vi "PPL_DRIVE_Get_Wheel_Speeds.vi"() -> (1 "Right Wheel Speed M/S":dbl format="%17.2f", 3 "Left Wheel Speed M/S":dbl format="%17.2f")   [LabVIEW 2019]
uses:
  PPL_DRIVE_GLOBALS.vi
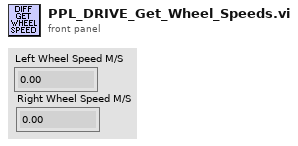
[diagram p1: front panel]
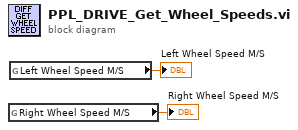
[diagram p0: block diagram]
diagram:
  n1 = global read "PPL_DRIVE_GLOBALS.vi" "Right Wheel Speed M/S"() -> (→"Right Wheel Speed M/S":dbl)
  n2 = global read "PPL_DRIVE_GLOBALS.vi" "Left Wheel Speed M/S"() -> (→"Left Wheel Speed M/S":dbl)
